vi "Sim Lidar.vi"() -> ()   [LabVIEW 2012]
uses:
  <vilib>/Platform/TimedLoop/XDataNode/timing_clust.ctl
  <vilib>/Platform/TimedLoop/XDataNode/nitl_modes.ctl
  <vilib>/Platform/TimedLoop/XDataNode/wakeup.ctl
  <instrlib>/Hokuyo URG Series/HAIOL/Hokuyo URG Series.lvclass
  <vilib>/Platform/TimedLoop/XDataNode/XDataNode.xnode
  <vilib>/Platform/TimedLoop/XDataNode/XDNodeRunTimeDep.lvlib
  <instrlib>/Hokuyo URG Series/HAIOL/Simulator/Hokuyo URG Series Simulator.lvclass
panel:
  in  "error in":errorcluster
  out "error out":errorcluster
  out "LIDAR Data":cluster{"Magnitude":dbl[], "Direction":dbl[]}
  in  "stop?":bool
  in  "start point (-135°)":dbl=-135.0
  in  "end point (135°)":dbl=135.0
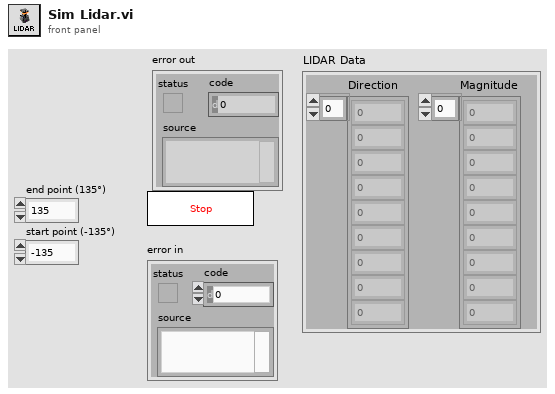
[diagram p1: front panel]
types:
  T1 = cluster{"Robot":string, "Sensors":string[], "Joints":string[], "Actuators":string[], "Robot Components":string[]}[]
  T2 = cluster{"Robot":string, "Sensors":string[], "Joints":string[], "Actuators":string[], "Robot Components":string[]}
  T3 = typedef "XDNodeRunTimeDep.lvlib/timing_clust.ctl" = cluster{"Expected End [f-1]":u64, "Actual End [f-1]":u64, "Finished Late? [f-1]":bool, "Expected End [i-1]":u64, "Actual End [i-1]":u64, "Finished Late? [i-1]":bool, "Expected Start [i]":u64, "Actual Start [i]":u64, "Expected Start [f]":u64, "Actual Start [f]":u64, "Source Name":string, "Structure Name":string, "Period":i64, "Deadline":i64, "Offset":i64, "Start":i64, "Priority":i32, "Timeout":i32, "Mode":T4, "Wakeup Reason":T5, "Error":errorcluster, "Source Type":string, "Secondary Source Type":string, "Global End Time":u64, "Global Start Time":u64, "Frame Duration":u64, "Iteration Duration":u64, "Assigned CPU":i32, "I/O Scan Engine Mode":u32}
  T4 = typedef "XDNodeRunTimeDep.lvlib/nitl_modes.ctl" = enum32{"No Change", "Process missed periods, maintain original phase", "Discard missed periods, maintain original phase", "Process missed periods, ignore original phase", "Discard missed periods, ignore original phase"}
  T5 = typedef "XDNodeRunTimeDep.lvlib/wakeup.ctl" = enum32{"Normal", "Aborted", "Asynchronous wakeup", "Timing source error", "Timed loop error", "Timeout"}
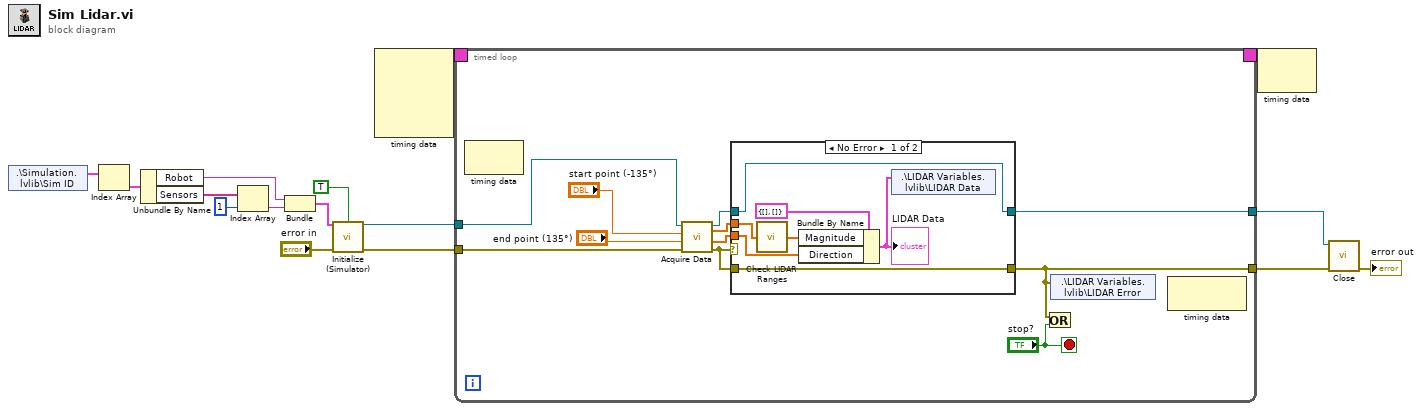
[diagram p0: block diagram]
diagram:
  n1 = shared-variable ".\\Simulation.lvlib\\Sim ID"() -> (w9:T1)  [unwired: 1 in, 1 out]
  n2 = Index Array(array=w9) -> (element=w8:T2)  [unwired: 1 in]
  n3 = Unbundle By Name(w8) -> ("Robot"=w4:string, "Sensors"=w7:string[])
  n4 = Index Array(array=w7, index=1) -> (element=w5:string)
  n5 = Bundle("Robot"=w4, w5) -> (w3:cluster{"Robot":string, string})  [unwired: 1 in]
  n6 = call <instrlib>:"Initialize (Simulator).vi"("Device ID"=w3, "Reset? (F: No)"=TRUE, "error in (no error)"="error in") -> ("Hokuyo URG Series out"=w1:refnum<class "Hokuyo URG Series.lvclass">, "error out"=w14:errorcluster)  [unwired: 11 in]
  n7 = node-c288() -> (w16:T3)  [unwired: 4 out]
  n8 = timed-loop {
    timing: w16 -> [_]
    timing-out: [_] -> w15
    tunnel: w1 -> [w24]
    tunnel: [w27] -> w11
    tunnel: [w26] -> w12
    tunnel: w14 -> [w23]
    stop <- "stop?" stop-if-true
    n9 = node-c288() -> ()  [unwired: 2 out]
    n10 = call-dynamic "Acquire Data.vi"("error in (no error)"=w23, "End Point (120 deg)"="end point (135°)", "Start Point (-120 deg)"="start point (-135°)", "Hokuyo URG Series in"=w24) -> ("error out"=w22:errorcluster, "Direction"=w19:dbl[], "Magnitude"=w20:dbl[], "Hokuyo URG Series out"=w21:refnum<class "Hokuyo URG Series.lvclass">)  [unwired: 4 in]
    n11 = case shown="No Error" w22 {
      selector: w22 -> [_ w35]
      tunnel: w20 -> [w28 _]
      tunnel: w19 -> [w31 _]
      tunnel: w21 -> [w34 w36]
      tunnel: [w34 w36] -> w27
      tunnel: [w33 w35] -> w26
      tunnel: w22 -> [w33 _]
      frame No Error {
        n12 = call "Check LIDAR Ranges.vi"("Magnitude"=w28) -> ("Magnitude out"=w29:dbl[])  [unwired: 4 in]
        n13 = Bundle By Name(cluster=cluster{"Magnitude":dbl[], "Direction":dbl[]} {"Magnitude"=[], "Direction"=[]} ("LIDAR Data"), "Magnitude"=w29, "Direction"=w31) -> (w30:cluster{"Magnitude":dbl[], "Direction":dbl[]})
        "LIDAR Data" <- w30
        n14 = shared-variable ".\\LIDAR Variables.lvlib\\LIDAR Data"(w30) -> ()  [unwired: 1 in, 1 out]
      }
      frame Error {
      }
    }
    n15 = Or(x=w26, y="stop?") -> ()  [unwired: 1 out]
    n16 = shared-variable ".\\LIDAR Variables.lvlib\\LIDAR Error"(w26) -> ()  [unwired: 1 in, 1 out]
    n17 = node-c288() -> ()  [unwired: 2 out]
  }
  n18 = node-c288(w15) -> ()  [unwired: 1 out]
  n19 = call-dynamic "Close.vi"("error in (no error)"=w12, "Hokuyo URG Series in"=w11) -> ("error out"=→"error out":errorcluster)  [unwired: 9 in]
